vi "OAT Tachless Limit of Mask Orders.vi"(6 "Time Boundary":cluster{"Time 1":dbl, "Time 2":dbl} {"Time 2" format="%.2f"; "Time 1" format="%.2f"}, 9 "bandwidth":T1={"bandwidth value"=0.5, "bandwidth unit"=enum."Order"} {"bandwidth value" min=0.0 format="%.2f"}, 10 "reference orders":dbl[](array[numeric]) format="%.2f", 11 "speed profile":T2 {"speed [RPM]" format="%.2f"; "time [s]" format="%.2f"}) -> (2 "lower limits":cluster{"time [s]":dbl[], "limit [Hz]":dbl[]}[](array[cluster]) {"limit [Hz]" format="%.2f"; "time [s]" format="%.2f"}, 3 "upper limits":cluster{"time [s]":dbl[], "limit [Hz]":dbl[]}[](array[cluster]) {"limit [Hz]" format="%.2f"; "time [s]" format="%.2f"})   [LabVIEW 2017, in "SoundVib_Tachless.lvlib"]
uses:
  <vilib>/addons/Sound and Vibration/Order Analysis/Tachless/SoundVib_Tachless.lvlib
  <vilib>/addons/Sound and Vibration/Order Analysis/Tach Process/SubVIs/speed profile.ctl
  <vilib>/addons/Sound and Vibration/Order Analysis/Ref Gabor Order Tracking/Mask Bandwidth.ctl
  <vilib>/addons/Sound and Vibration/Order Analysis/Tach Process/SoundVib_TachProcess.lvlib
  <vilib>/addons/Sound and Vibration/Order Analysis/Gabor Order Tracking/SoundVib_Gabor.lvlib
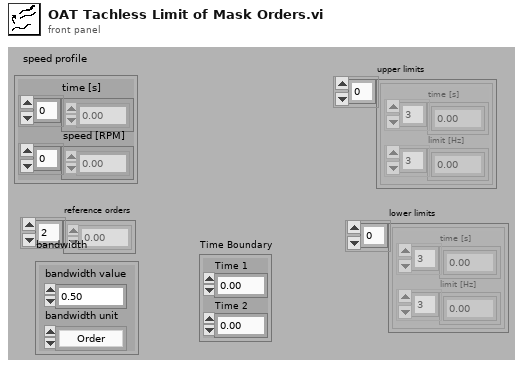
[diagram p1: front panel]
types:
  T1 = typedef "SoundVib_Gabor.lvlib/Mask Bandwidth.ctl" = cluster{"bandwidth value":dbl, "bandwidth unit":enum16{"Order", "Hz"}}
  T2 = typedef "SoundVib_TachProcess.lvlib/speed profile.ctl" = cluster{"time [s]":dbl[], "speed [RPM]":dbl[]}
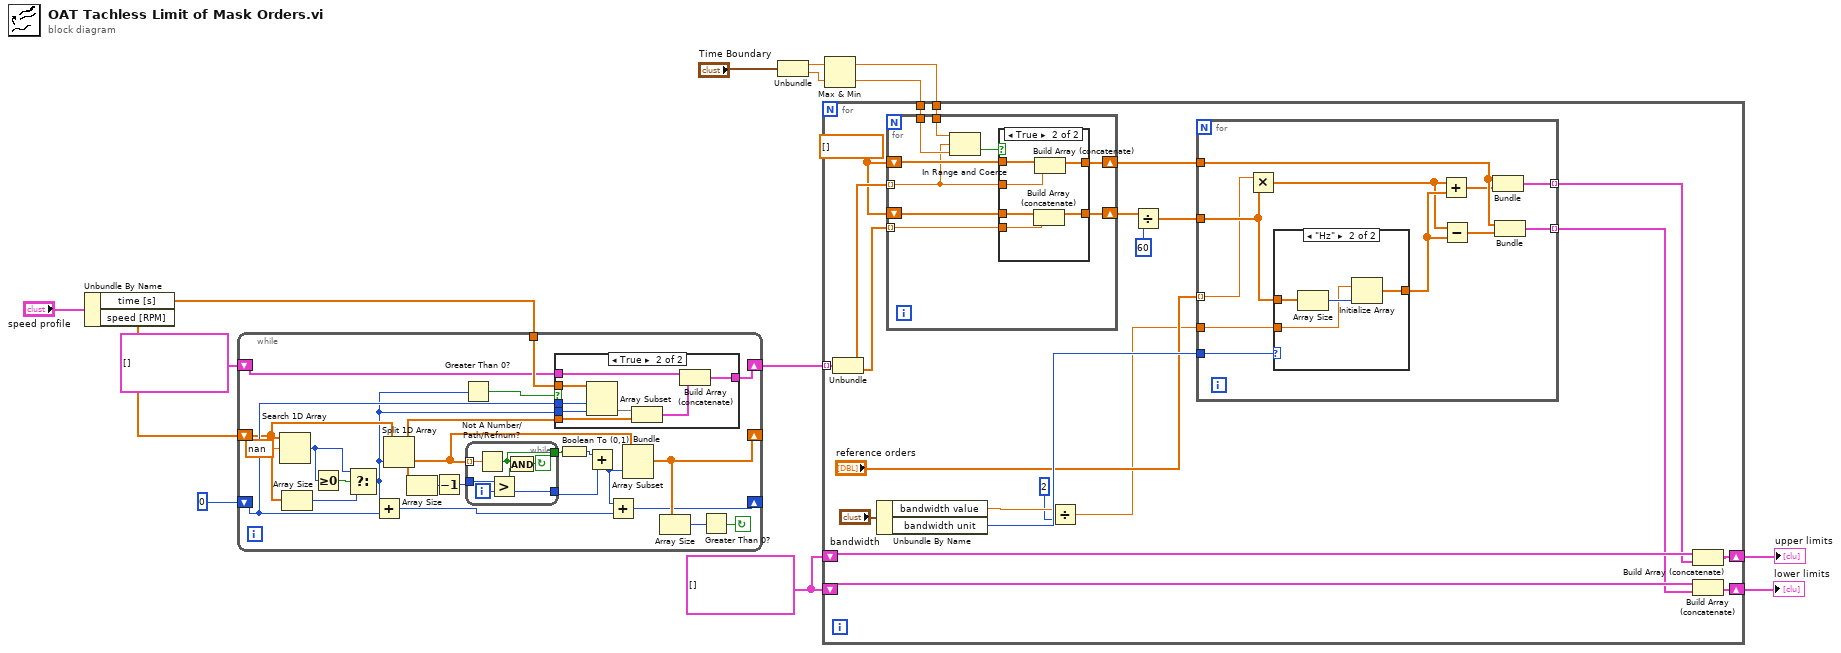
[diagram p0: block diagram]
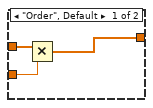
[diagram p4: hidden frame]
diagram:
  w1 = cluster{dbl[], dbl[]}[] []
  n1 = Unbundle By Name("speed profile") -> ("time [s]"=w12:dbl[], "speed [RPM]"=w11:dbl[])
  n2 = while {
    shift-left: cluster{dbl[], dbl[]}[] [] -> [w16]
    shift-right: [w17] -> w8
    tunnel: w12 -> [w34]
    shift-left: 0 -> [w33]
    shift-right: [w27] -> _
    shift-left: w11 -> [w24]
    shift-right: [w28] -> _
    stop <- w36 continue-if-true
    n3 = Search 1D Array(1D array=w24, element=nan) -> (index of element=w25:i32)  [unwired: 1 in]
    n4 = Array Size(array=w24) -> (size(s)=w23:i32)
    n5 = Greater Or Equal To 0?(x=w25) -> (x >= 0?=w26:bool)
    n6 = Select(t=w25, s=w26, f=w23) -> (s? t:f=w18:i32)
    n7 = Add(x=w18, y=w33) -> (x+y=w35:i32)
    n8 = Split 1D Array(array=w24, index=w18) -> (first subarray=w32:dbl[], second subarray=w29:dbl[])
    n9 = Array Size(array=w29) -> (size(s)=w31:i32)
    n10 = Decrement(x=w31) -> (x-1=w30:i32)
    n11 = Greater Than 0?(x=w18) -> (x > 0?=w15:bool)
    n12 = while {
      tunnel: [w39] -> w22
      tunnel: [w42] -> w20
      tunnel: w30 -> [w43]
      tunnel: w29 -> [w44] mode=indexing
      i -> [w42]
      stop <- w40 continue-if-true
      n13 = Not A Number/Path/Refnum?(number/path/refnum=w44) -> (NaN/Path/Refnum?=w39:bool)
      n14 = Greater?(x=w43, y=w42) -> (0:w41:bool)
      n15 = And(x=w39, y=w41) -> (x .and. y?=w40:bool)
    }
    n16 = case shown="True" w15 {
      tunnel: w34 -> [_ w53]
      tunnel: w33 -> [_ w52]
      tunnel: w32 -> [_ w50]
      tunnel: w18 -> [_ w49]
      tunnel: [w45 w47] -> w17
      tunnel: w16 -> [w45 w46]
      frame False {
      }
      frame True {
        n17 = Array Subset(array=w53, index=w52, length=w49) -> (w51:dbl[])
        n18 = Bundle(w51, w50) -> (w48:cluster{dbl[], dbl[]})  [unwired: 1 in]
        n19 = Build Array (concatenate)(w46, w48) -> (w47:cluster{dbl[], dbl[]}[])
      }
    }
    n20 = Boolean To (0,1)(Boolean=w22) -> (0, 1=w21:i16)
    n21 = Add(x=w21, y=w20) -> (x+y=w19:i32)
    n22 = Add(x=w19, y=w35) -> (x+y=w27:i32)
    n23 = Array Subset(array=w29, index=w19) -> (w28:dbl[])  [unwired: 1 in]
    n24 = Array Size(array=w28) -> (size(s)=w37:i32)
    n25 = Greater Than 0?(x=w37) -> (x > 0?=w36:bool)
  }
  n26 = Unbundle("Time Boundary") -> ("Time 1"=w5:dbl, "Time 2"=w4:dbl)
  n27 = Max & Min(x=w5, y=w4) -> (max(x,y)=w3:dbl, min(x,y)=w2:dbl)
  n28 = for {
    tunnel: w8 -> [w67] mode=indexing
    shift-right: [w65] -> w10
    shift-left: w1 -> [w66]
    shift-right: [w64] -> w9
    shift-left: w1 -> [w63]
    tunnel: w3 -> [w60]
    tunnel: w2 -> [w59]
    w55 = dbl[] []
    n29 = Unbundle(w67) -> (w58:dbl[], w56:dbl[])
    n30 = Unbundle By Name("bandwidth") -> ("bandwidth value"=w72:dbl, "bandwidth unit"=w74:enum16{"Order", "Hz"})
    n31 = for {
      shift-right: [w84] -> w57
      shift-left: w55 -> [w83]
      tunnel: w58 -> [w77] mode=indexing
      tunnel: w56 -> [w81] mode=indexing
      shift-right: [w80] -> w54
      shift-left: w55 -> [w82]
      tunnel: w60 -> [w79]
      tunnel: w59 -> [w78]
      n32 = In Range and Coerce(upper limit=w79, x=w77, lower limit=w78) -> (In Range?=w76:bool)  [unwired: 1 out]
      n33 = case shown="True" w76 {
        tunnel: [w86 w92] -> w84
        tunnel: w83 -> [w86 w91]
        tunnel: w82 -> [w85 w90]
        tunnel: w81 -> [_ w89]
        tunnel: [w85 w88] -> w80
        tunnel: w77 -> [_ w87]
        frame False {
        }
        frame True {
          n34 = Build Array (concatenate)(w90, w89) -> (w88:dbl[])
          n35 = Build Array (concatenate)(w91, w87) -> (w92:dbl[])
        }
      }
    }
    n36 = Divide(x=w72, y=2) -> (x/y=w69:dbl)
    n37 = Divide(x=w54, y=60) -> (x/y=w70:dbl[])
    n38 = for {
      tunnel: w74 -> [w103]
      tunnel: w69 -> [w102]
      tunnel: "reference orders" -> [w95] mode=indexing
      tunnel: w70 -> [w96]
      tunnel: [w101] -> w62 mode=indexing
      tunnel: [w100] -> w61 mode=indexing
      tunnel: w57 -> [w99]
      n39 = Multiply(x=w95, y=w96) -> (x*y=w93:dbl[])
      n40 = case shown="\"Hz\"" w103 {
        tunnel: [w105 w107] -> w94
        tunnel: w102 -> [w104 w108]
        tunnel: w96 -> [w106 w110]
        frame "Order", Default {
          n41 = Multiply(x=w106, y=w104) -> (x*y=w105:dbl[])
        }
        frame "Hz" {
          n42 = Array Size(array=w110) -> (size(s)=w109:i32)
          n43 = Initialize Array(w108, w109) -> (w107:dbl[])
        }
      }
      n44 = Add(x=w93, y=w94) -> (x+y=w98:dbl[])
      n45 = Subtract(x=w93, y=w94) -> (x-y=w97:dbl[])
      n46 = Bundle(w99, w98) -> (w101:cluster{dbl[], dbl[]})  [unwired: 1 in]
      n47 = Bundle(w99, w97) -> (w100:cluster{dbl[], dbl[]})  [unwired: 1 in]
    }
    n48 = Build Array (concatenate)(w66, w62) -> (w65:cluster{dbl[], dbl[]}[])
    n49 = Build Array (concatenate)(w63, w61) -> (w64:cluster{dbl[], dbl[]}[])
  }
  "upper limits" <- w10
  "lower limits" <- w9
